vi "Kaelus PIM Manage PIMHW Connection Daemon.vi"(6 "Disconnect TCP? (f)":bool, 7 "Session Conn Cmd":T3=enum."KEEP_ALIVE", 8 "error in (no error)":errorcluster, 10 "PIM Config (Connection only)":T1={"host IP (localhost)"="localhost", "host Port"=3388, "Model"="", "Serial Number(s)"="", "Calibration Date"=3388.0, "Dual Port?"=FALSE, "DeviceNames"=[], "Parameters"={"TX1start"=0.0, "TX1stop"=0.0, "TX1pmax"=0.0, "TX2start"=0.0, "TX2stop"=0.0, "TX2pmax"=0.0, "RXstart"=0.0, "RXstop"=0.0}, "Interface"=enum."PIM Web Engine"} {"Calibration Date" format="%.2f"; "Parameters"."TX2pmax" format="%.1f"; "Parameters"."TX1pmax" format="%.1f"; "Parameters"."RXstop" format="%.1f"; "Parameters"."RXstart" format="%.1f"; "Parameters"."TX2stop" format="%.1f"; "Parameters"."TX2start" format="%.1f"; "Parameters"."TX1stop" format="%.1f"; "Parameters"."TX1start" format="%.1f"}, 11 "daemon ref":refnum<vi>) -> (0 "error out":errorcluster, 3 "daemon ref out":refnum<vi>)   [LabVIEW 2011]
uses:
  TypeDefs/Kaelus PIM PIMHW Connection CMDS.ctl
  PIM Configuration.ctl
  PIM Interface Language.ctl
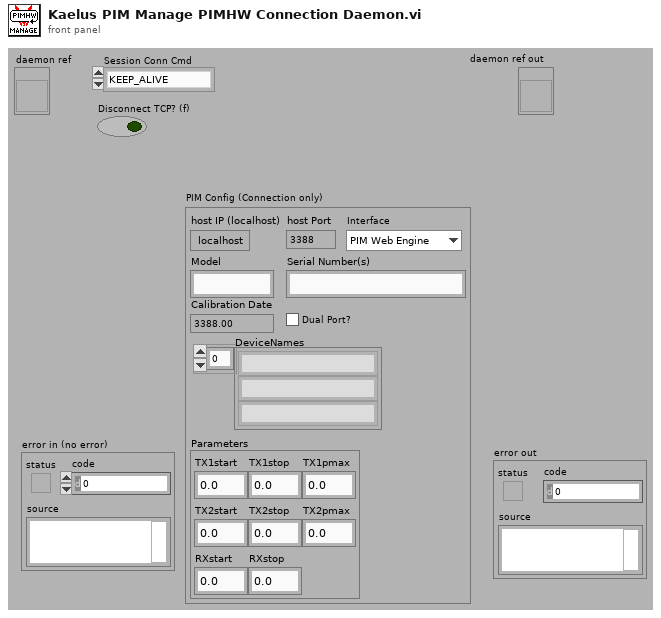
[diagram p1: front panel]
types:
  T1 = typedef "PIM Configuration.ctl" = cluster{"host IP (localhost)":string, "host Port":u16, "Model":string, "Serial Number(s)":string, "Calibration Date":dbl, "Dual Port?":bool, "DeviceNames":string[], "Parameters":cluster{"TX1start":dbl, "TX1stop":dbl, "TX1pmax":dbl, "TX2start":dbl, "TX2stop":dbl, "TX2pmax":dbl, "RXstart":dbl, "RXstop":dbl}, "Interface":T2}
  T2 = typedef "PIM Interface Language.ctl" = enum16{"PIM Web Engine", "PIM HW Engine"}
  T3 = typedef "Kaelus PIM PIMHW Connection CMDS.ctl" = enum16{"CONNECT", "DISCONNECT", "KEEP_ALIVE"}
  T4 = enum32{"Bad", "Idle", "Run top level", "Running"}
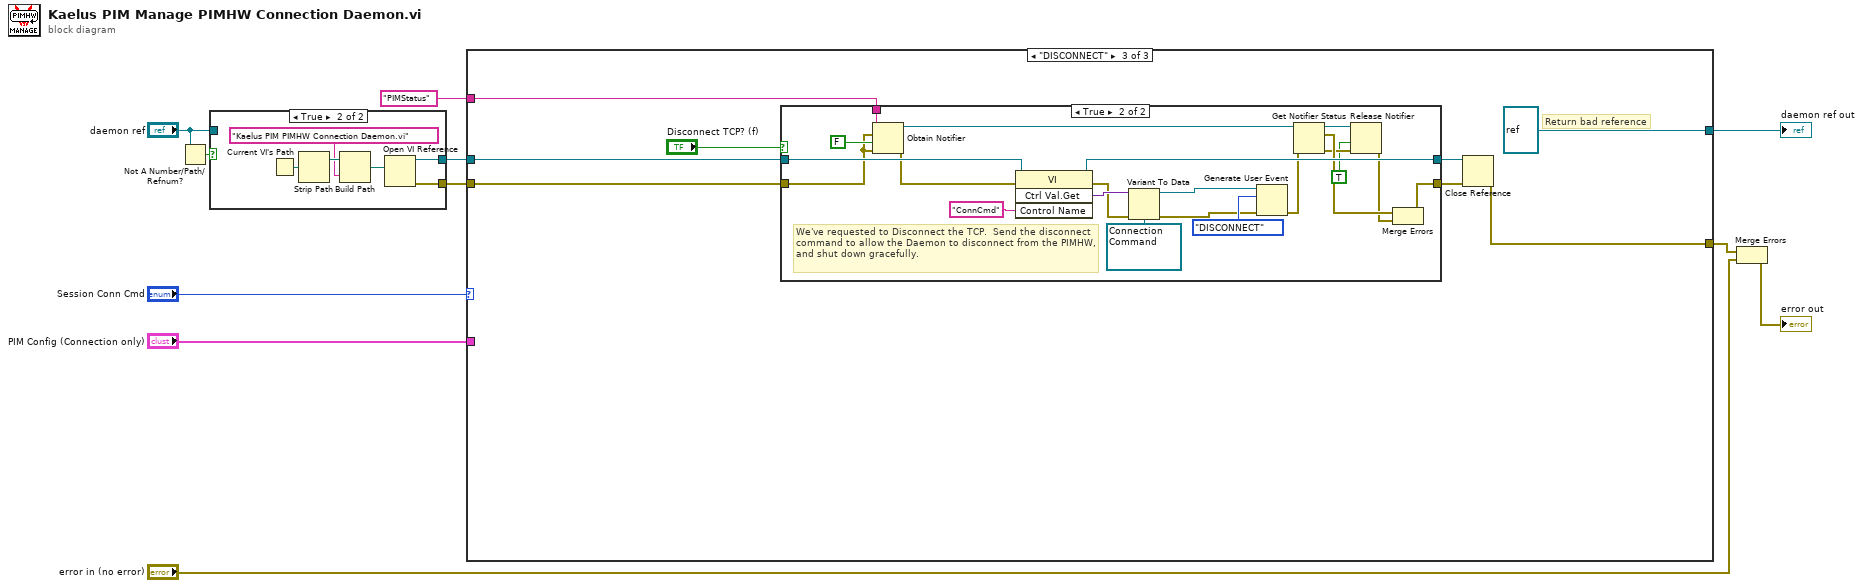
[diagram p0: block diagram]
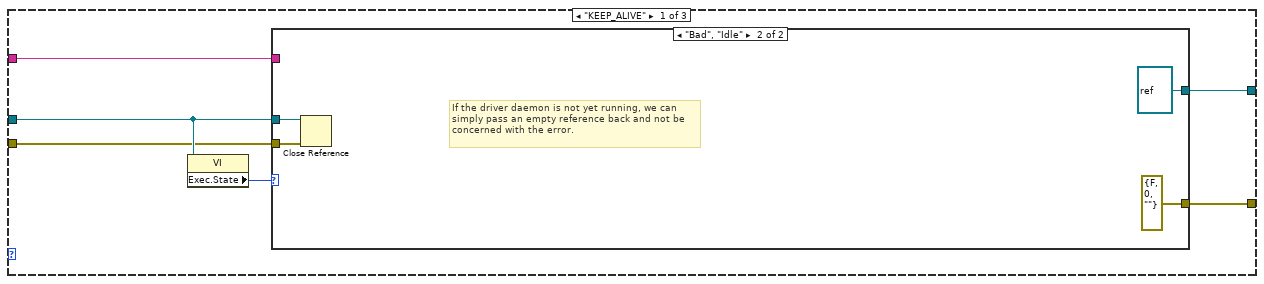
[diagram p2: hidden frame]
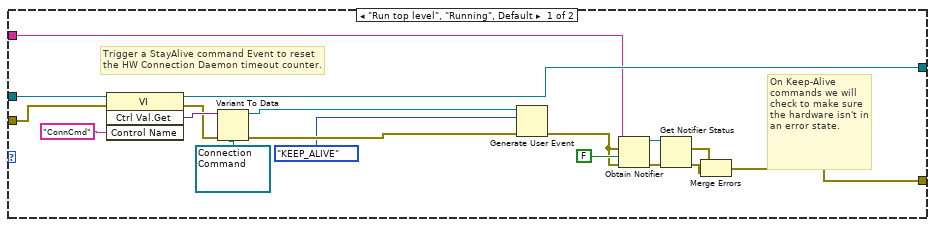
[diagram p3: hidden frame]
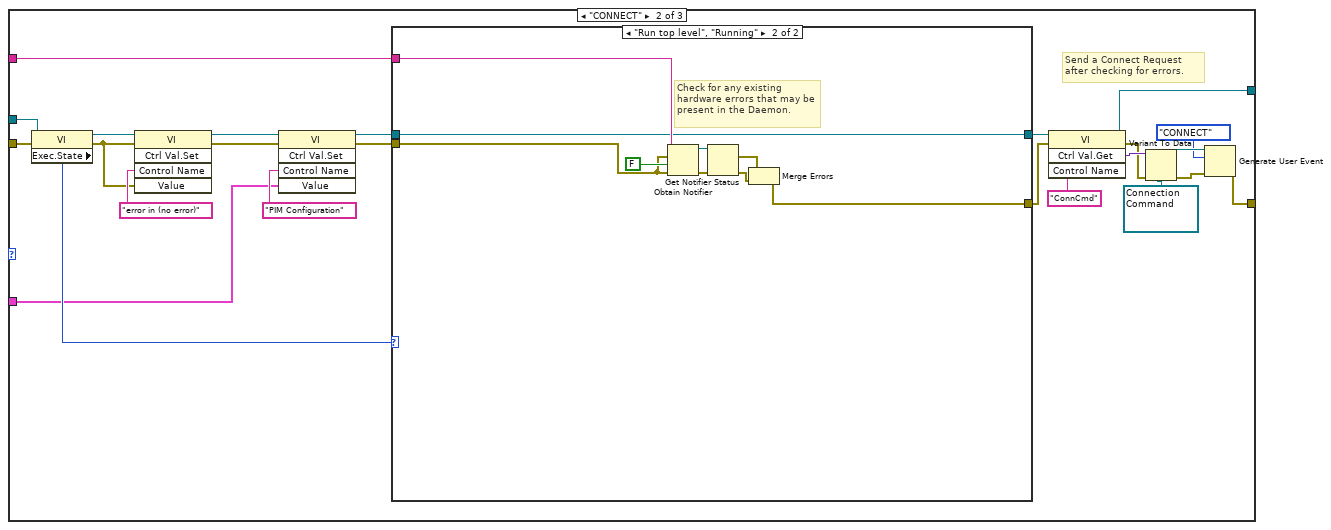
[diagram p4: hidden frame]
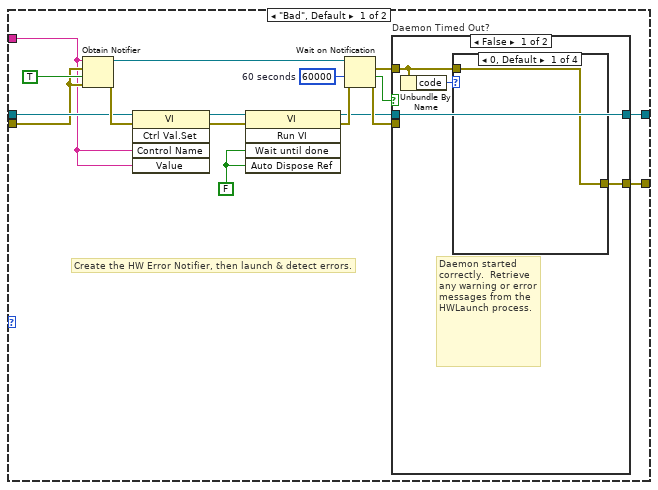
[diagram p5: hidden frame]
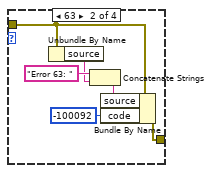
[diagram p6: hidden frame]
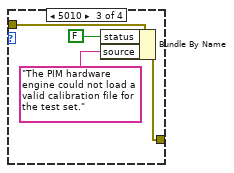
[diagram p7: hidden frame]
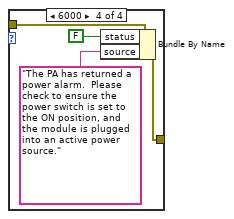
[diagram p8: hidden frame]
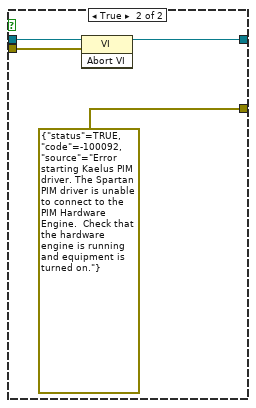
[diagram p9: hidden frame]
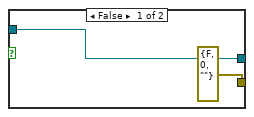
[diagram p11: hidden frame]
diagram:
  n1 = Not A Number/Path/Refnum?(number/path/refnum="daemon ref") -> (NaN/Path/Refnum?=w9:bool)
  n2 = case shown="True" w9 {
    tunnel: [w13 w16] -> w11
    tunnel: [errorcluster {"status"=FALSE, "code"=0, "source"=""} ("error out") w15] -> w10
    tunnel: "daemon ref" -> [w13 _]
    frame False {
    }
    frame True {
      n3 = Current VI's Path() -> (path=w18:path)
      n4 = Strip Path(path=w18) -> (stripped path=w17:path)  [unwired: 1 out]
      n5 = Build Path(base path=w17, name or relative path="Kaelus PIM PIMHW Connection Daemon.vi") -> (appended path=w19:path)
      n6 = Open VI Reference(vi path=w19) -> (vi reference=w16:refnum<vi>, error out=w15:errorcluster)  [unwired: 1 in, 4 out]
    }
  }
  n7 = case shown="\"DISCONNECT\"" "Session Conn Cmd" {
    tunnel: w11 -> [w22 w71 w126]
    tunnel: w10 -> [w21 w70 w123]
    tunnel: [w23 w53 w127] -> w4
    tunnel: [w25 w52 refnum<vi> refnum] -> w7
    tunnel: "PIMStatus" ("Control Name") -> [w24 w54 w122]
    tunnel: "PIM Config (Connection only)" -> [_ w50 _]
    frame "KEEP_ALIVE" {
      n8 = property class="VI"(reference=w22) -> ("Exec.State"=w20:T4)  [unwired: 1 in, 2 out]
      n9 = case shown="\"Bad\", \"Idle\"" w20 {
        tunnel: w22 -> [w36 w44]
        tunnel: [w35 refnum<vi> refnum ("daemon ref")] -> w25
        tunnel: w24 -> [w33 _]
        tunnel: [w31 errorcluster {"status"=FALSE, "code"=0, "source"=""} ("error out")] -> w23
        tunnel: w21 -> [w26 w45]
        frame "Run top level", "Running", Default {
          w40 = refnum<user-event> refnum items=["CONNECT", "DISCONNECT", "KEEP_ALIVE"] ("ConnCmd")
          # "On Keep-Alive commands we will check to make sure the hardware isn't in an error state."
          # "Trigger a StayAlive command Event to reset the HW Connection Daemon timeout counter."
          n10 = invoke class="VI" method="Ctrl Val.Get"(reference=w36, error in=w26, "Control Name"="ConnCmd") -> (reference out=w35:refnum<vi>, error out=w41:errorcluster, "Get Control Value Variant"=w42:variant)  [unwired: 1 in, 1 out]
          n11 = Variant To Data(error in=w41, type=w40, Variant=w42) -> (data=w39:refnum<user-event>, error out=w38:errorcluster)
          n12 = Generate User Event(user event=w39, event data cluster=Kaelus_PIM_PIMHW_Connection_CMDS."KEEP_ALIVE" ("Connection Command"), error in=w38) -> (error out=w32:errorcluster)  [unwired: 1 out]
          n13 = Obtain Notifier(name (unnamed)=w33, notification data type=w32, create if not found? (T)=FALSE, error in (no error)=w32) -> (notifier out=w30:refnum<notifier>, error out=w29:errorcluster)  [unwired: 1 out]
          n14 = Get Notifier Status(notifier=w30, error in (no error)=w29) -> (current notification=w27:errorcluster, error out=w28:errorcluster)  [unwired: 3 out]
          n15 = Merge Errors(w27, w28) -> (w31:errorcluster)
        }
        frame "Bad", "Idle" {
          # "If the driver daemon is not yet running, we can simply pass an empty reference back and not be concerned with the error."
          n16 = Close Reference(reference=w44, error in (no error)=w45) -> ()  [unwired: 1 out]
        }
      }
    }
    frame "CONNECT" {
      w60 = refnum<user-event> refnum items=["CONNECT", "DISCONNECT", "KEEP_ALIVE"] ("ConnCmd")
      # "Send a Connect Request after checking for errors."
      n17 = property class="VI"(reference=w71, error in=w70) -> (reference out=w56:refnum<vi>, error out=w55:errorcluster, "Exec.State"=w51:T4)
      n18 = invoke class="VI" method="Ctrl Val.Set"(reference=w56, error in=w55, "Control Name"="error in (no error)", "Value"=w55) -> (reference out=w68:refnum<vi>, error out=w67:errorcluster)  [unwired: 1 in, 3 out]
      n19 = invoke class="VI" method="Ctrl Val.Set"(reference=w68, error in=w67, "Control Name"="PIM Configuration", "Value"=w50) -> (reference out=w48:refnum<vi>, error out=w49:errorcluster)  [unwired: 1 in, 3 out]
      n20 = case shown="\"Run top level\", \"Running\"" w51 {
        tunnel: w48 -> [w74 w113]
        tunnel: [w76 w118] -> w65
        tunnel: w49 -> [w73 w112]
        tunnel: [w79 w113] -> w64
        tunnel: w54 -> [w72 w120]
        frame "Bad", Default {
          w83 = 60000  # 60 seconds
          w84 = FALSE ("Wait Until Done")
          # "Create the HW Error Notifier, then launch & detect errors."
          n21 = Obtain Notifier(name (unnamed)=w72, notification data type=w73, create if not found? (T)=TRUE ("Wait Until Done"), error in (no error)=w73) -> (notifier out=w88:refnum<notifier>, error out=w75:errorcluster)  [unwired: 1 out]
          n22 = invoke class="VI" method="Ctrl Val.Set"(reference=w74, error in=w75, "Control Name"=w72, "Value"=w72) -> (reference out=w86:refnum<vi>, error out=w87:errorcluster)  [unwired: 1 in, 3 out]
          n23 = invoke class="VI" method="Run VI"(reference=w86, error in=w87, "Wait until done"=w84, "Auto Dispose Ref"=w84) -> (reference out=w80:refnum<vi>, error out=w85:errorcluster)  [unwired: 1 in, 3 out]
          n24 = Wait on Notification(notifier=w88, timeout in ms (-1)=w83, error in (no error)=w85) -> (notification=w77:errorcluster, timed out?=w82:bool, error out=w81:errorcluster)  [unwired: 2 out]
          n25 = case "Daemon Timed Out?" shown="False" w82 {
            tunnel: w81 -> [_ w111]
            tunnel: w80 -> [w92 w110]
            tunnel: [w92 w109] -> w79
            tunnel: [w89 errorcluster {"status"=TRUE, "code"=-100092, "source"="Error starting Kaelus PIM driver. The Spartan PIM driver is unable to connect to the PIM Hardware Engine.  Check that the hardware engine is running and equipment is turned on."} ("error out")] -> w76
            tunnel: w77 -> [w90 _]
            frame False {
              # "Daemon started correctly.  Retrieve any warning or error messages from the HWLaunch process."
              n26 = Unbundle By Name(w90) -> ("code"=w91:i32)
              n27 = case shown="0, Default" w91 {
                tunnel: w90 -> [w93 w98 w103 w107]
                tunnel: [w93 w94 w100 w104] -> w89
                frame 0, Default {
                }
                frame 63 {
                  n28 = Unbundle By Name(w98) -> ("source"=w96:string)
                  n29 = Concatenate Strings("Error 63: " ("string"), w96) -> (w95:string)
                  n30 = Bundle By Name(cluster=w98, "source"=w95, "code"=-100092) -> (w94:errorcluster)
                }
                frame 5010 {
                  n31 = Bundle By Name(cluster=w103, "status"=FALSE, "source"="The PIM hardware engine could not load a valid calibration file for the test set." ("Control Name")) -> (w100:errorcluster)
                }
                frame 6000 {
                  n32 = Bundle By Name(cluster=w107, "status"=FALSE, "source"="The PA has returned a power alarm.  Please check to ensure the power switch is set to the ON position, and the module is plugged into an active power source." ("Control Name")) -> (w104:errorcluster)
                }
              }
            }
            frame True {
              n33 = invoke class="VI" method="Abort VI"(reference=w110, error in=w111) -> (reference out=w109:refnum<vi>)  [unwired: 1 in, 2 out]
            }
          }
        }
        frame "Run top level", "Running" {
          # "Check for any existing hardware errors that may be present in the Daemon."
          n34 = Obtain Notifier(name (unnamed)=w120, notification data type=w112, create if not found? (T)=FALSE, error in (no error)=w112) -> (notifier out=w117:refnum<notifier>, error out=w116:errorcluster)  [unwired: 1 out]
          n35 = Get Notifier Status(notifier=w117, error in (no error)=w116) -> (current notification=w115:errorcluster, error out=w114:errorcluster)  [unwired: 3 out]
          n36 = Merge Errors(w115, w114) -> (w118:errorcluster)
        }
      }
      n37 = invoke class="VI" method="Ctrl Val.Get"(reference=w64, error in=w65, "Control Name"="ConnCmd") -> (reference out=w52:refnum<vi>, error out=w61:errorcluster, "Get Control Value Variant"=w62:variant)  [unwired: 1 in, 1 out]
      n38 = Variant To Data(error in=w61, type=w60, Variant=w62) -> (data=w59:refnum<user-event>, error out=w58:errorcluster)
      n39 = Generate User Event(user event=w59, event data cluster=Kaelus_PIM_PIMHW_Connection_CMDS."CONNECT" ("Connection Command"), error in=w58) -> (error out=w53:errorcluster)  [unwired: 1 out]
    }
    frame "DISCONNECT" {
      # "Return bad reference"
      n40 = case shown="True" "Disconnect TCP? (f)" {
        tunnel: w126 -> [w130 w144]
        tunnel: w123 -> [w129 w138]
        tunnel: [w130 w143] -> w124
        tunnel: w122 -> [_ w140]
        tunnel: [w129 w139] -> w121
        frame False {
          # "Unless we've specifically commanded the TCP to be disconnected, we will allow the Daemon thread to continue executing."
        }
        frame True {
          w148 = refnum<user-event> refnum items=["CONNECT", "DISCONNECT", "KEEP_ALIVE"] ("ConnCmd")
          # "We've requested to Disconnect the TCP.  Send the disconnect command to allow the Daemon to disconnect from the PIMHW, and shut down gracefully."
          n41 = Obtain Notifier(name (unnamed)=w140, notification data type=w138, create if not found? (T)=FALSE, error in (no error)=w138) -> (notifier out=w135:refnum<notifier>, error out=w137:errorcluster)  [unwired: 1 out]
          n42 = invoke class="VI" method="Ctrl Val.Get"(reference=w144, error in=w137, "Control Name"="ConnCmd") -> (reference out=w143:refnum<vi>, error out=w145:errorcluster, "Get Control Value Variant"=w147:variant)  [unwired: 1 in, 1 out]
          n43 = Variant To Data(error in=w145, type=w148, Variant=w147) -> (data=w149:refnum<user-event>, error out=w150:errorcluster)
          n44 = Generate User Event(user event=w149, event data cluster=Kaelus_PIM_PIMHW_Connection_CMDS."DISCONNECT" ("Connection Command"), error in=w150) -> (error out=w136:errorcluster)  [unwired: 1 out]
          n45 = Get Notifier Status(notifier=w135, error in (no error)=w136) -> (notifier out=w133:refnum<notifier>, current notification=w142:errorcluster, error out=w134:errorcluster)  [unwired: 2 out]
          n46 = Release Notifier(notifier=w133, force destroy? (F)=TRUE, error in (no error)=w134) -> (error out=w131:errorcluster)  [unwired: 2 out]
          n47 = Merge Errors(w142, w131) -> (w139:errorcluster)
        }
      }
      n48 = Close Reference(reference=w124, error in (no error)=w121) -> (error out=w127:errorcluster)
    }
  }
  "daemon ref out" <- w7
  n49 = Merge Errors(w4, "error in (no error)") -> (→"error out":errorcluster)
